vi "Counter - Read Encoder (Finite Clock).vi"() -> ()   [LabVIEW 2017]
doc: "本范例演示使用DAQmx设备采集有限缓冲编码器测量的方法。 本范例采用外部时钟，从而计数寄存器采样按固定间隔进行。 如不需要实现计数寄存器确定性采样，请参考不采用外部时钟的Counter - Read Encoder.vi范例。\n\n关于将信号连接至DAQ设备的方法，可参考设备文档。"
uses:
  <vilib>/Utility/error.llb/DialogType.ctl
  <vilib>/DAQmx/read.llb/DAQmx Read (Counter 1D DBL 1Chan NSamp).vi
  <vilib>/DAQmx/create/channels.llb/DAQmx Create Channel (CI-Position-Angular Encoder).vi
  <vilib>/DAQmx/configure/timing.llb/DAQmx Timing (Sample Clock).vi
  <vilib>/DAQmx/miscellaneous.llb/DAQmx Fill In Error Info.vi
  <resource>/objmgr/daqmx.rc
panel:
  in  "Z索引接线端":tag="PFI9"
  in  "启用Z索引":bool
  in  "脉冲每转":u32=24
  in  "B输入接线端":tag="PFI10"
  in  "输入接线端":tag="PFI8"
  in  "计数器":tag="Dev1/ctr0"
  in  "触发类型":enum32{"No Trigger", "Digital Arm Start"}(tab)
  in  "边沿":i32(ring)=10280 items=["上升"=10280, "下降"=10171]
  in  "数字触发源":tag
  out "采集数据":dbl[](array[numeric])
  in  "采样":i32=100
  in  "采样率":dbl=1000.0
  in  "采样时钟源":tag="PFI0"
  # "通道设置"
  # "采集数据"
  # "定时设置"
  # "触发设置"
  # "如需配置并使用触发/计数重置，必须先在上面选择相应的选项卡。  有些硬件不支持上述选项－更多信息见设备的相应文档。"
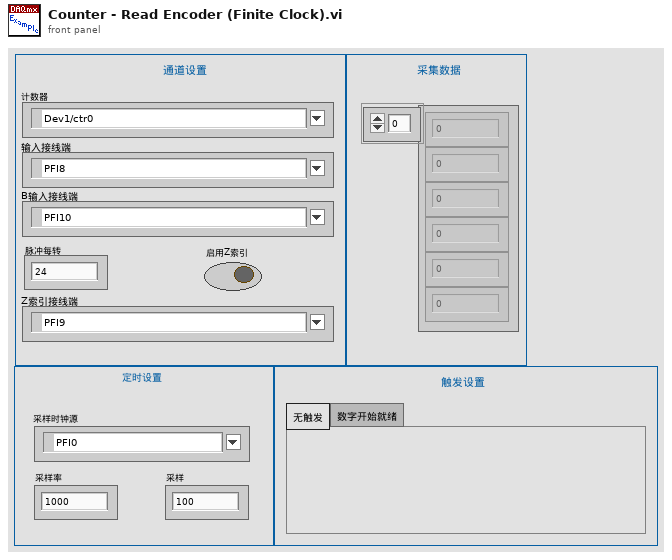
[diagram p1: front panel]
types:
  T1 = typedef "DialogType.ctl" = u16
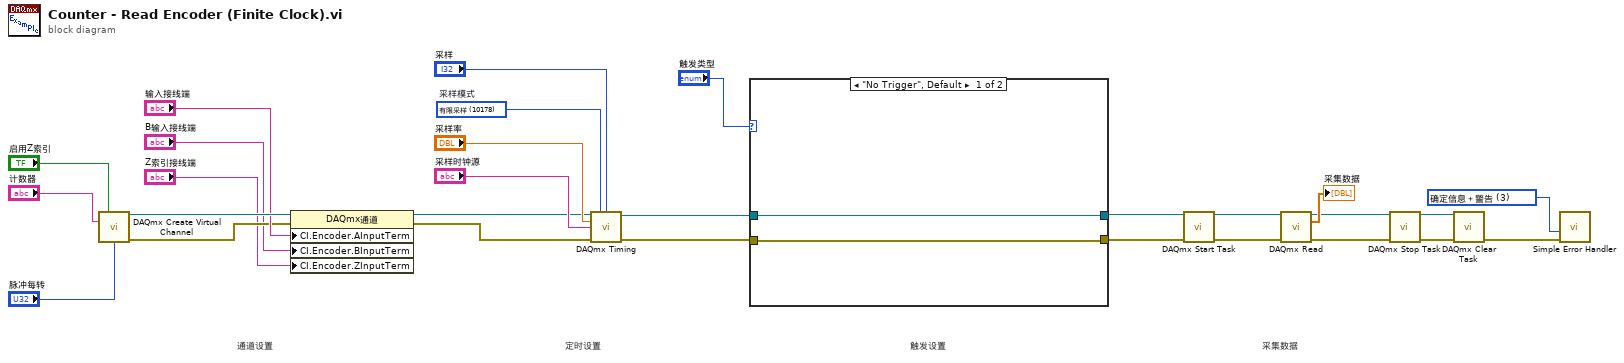
[diagram p0: block diagram]
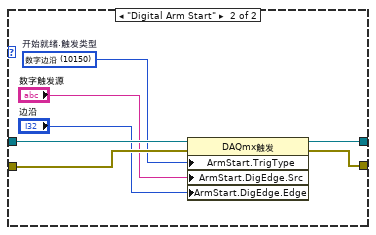
[diagram p2: hidden frame]
diagram:
  w1 = T1 3 items=["无对话框", "确定信息", "继续或停止信息", "确定信息＋警告", "继续/停止＋警告"] ("对话框类型（确定信息：1）")
  w28 = 10178 items=["有限采样"=10178, "连续采样"=10123, "硬件定时单点"=12522]  # 采样模式
  # "采集数据"
  # "触发设置"
  # "定时设置"
  # "通道设置"
  n1 = call-poly <vilib>:"DAQmx Create Virtual Channel.vi"("z index enable"="启用Z索引", "counter"="计数器", "pulses per revolution"="脉冲每转") -> ("task out"=w14:refnum<k21>, "error out"=w12:errorcluster)  [unwired: 11 in]
  n2 = property class="DAQmx通道"(reference=w14, error in=w12, "CI.Encoder.AInputTerm"="输入接线端", "CI.Encoder.BInputTerm"="B输入接线端", "CI.Encoder.ZInputTerm"="Z索引接线端") -> (reference out=w7:refnum<k21>, error out=w6:errorcluster)
  n3 = call-poly <vilib>:"DAQmx Timing.vi"("task/channels in"=w7, "sample mode"=w28, "samples per channel"="采样", "rate"="采样率", "source"="采样时钟源", "error in"=w6) -> ("task out"=w18:refnum<k21>, "error out"=w19:errorcluster)  [unwired: 8 in]
  n4 = case shown="\"No Trigger\", Default" "触发类型" {
    tunnel: w18 -> [w30 w37]
    tunnel: w19 -> [w29 w34]
    tunnel: [w30 w36] -> w16
    tunnel: [w29 w35] -> w17
    frame "No Trigger", Default {
    }
    frame "Digital Arm Start" {
      w31 = 10150 items=["数字边沿"=10150, "无"=10230]  # 开始就绪.触发类型
      n5 = property class="DAQmx触发"(reference=w37, error in=w34, "ArmStart.TrigType"=w31, "ArmStart.DigEdge.Src"="数字触发源", "ArmStart.DigEdge.Edge"="边沿") -> (reference out=w36:refnum<k21>, error out=w35:errorcluster)
    }
  }
  n6 = call <vilib>:"DAQmx Start Task.vi"("task/channels in"=w16, "error in"=w17) -> ("task out"=w27:refnum<k21>, "error out"=w26:errorcluster)  [unwired: 12 in]
  n7 = call-poly <vilib>:"DAQmx Read.vi"("task/channels in"=w27, "error in"=w26) -> ("task out"=w2:refnum<k21>, "data"=→"采集数据":dbl[], "error out"=w3:errorcluster)  [unwired: 11 in]
  n8 = call <vilib>:"DAQmx Stop Task.vi"("task/channels in"=w2, "error in"=w3) -> ("task out"=w4:refnum<k21>, "error out"=w5:errorcluster)  [unwired: 12 in]
  n9 = call <vilib>:"DAQmx Clear Task.vi"("task in"=w4, "error in"=w5) -> ("error out"=w25:errorcluster)  [unwired: 13 in]
  n10 = call <vilib>:"Simple Error Handler.vi"("type of dialog (OK msg:1)"=w1, "error in (no error)"=w25) -> ()  [unwired: 3 in, 5 out]
